vi "createFloat.vi"(8 "error in (no error)":errorcluster, 10 "Value":dbl, 11 "IInteger in":refnum<class "IFloat.lvclass">) -> (0 "error out":errorcluster, 3 "IInteger out":refnum<class "IFloat.lvclass">)   [LabVIEW 2022 SP3, in "openDAQ.lvlib" / "daqCoreTypes.lvlib" / "IFloat.lvclass"]
uses:
  <instrlib>/openDAQ/Public/Classes/daqCoreTypes/IFloat/IFloat.lvclass
  C:/Program Files (x86)/National Instruments/LabVIEW 2022/instr.lib/openDAQ/Public/Classes/IBaseObject/IBaseObject.lvclass
  <instrlib>/openDAQ/Public/Classes/IBaseObject/IBaseObject.lvclass/IBaseObject.ctl
  <instrlib>/openDAQ/Public/Classes/IBaseObject/Accessor/Read reference.vi
  <instrlib>/openDAQ/Public/Classes/IBaseObject/Accessor/Write reference.vi
  <instrlib>/openDAQ/Binaries/Windows/x86/copendaq32.dll
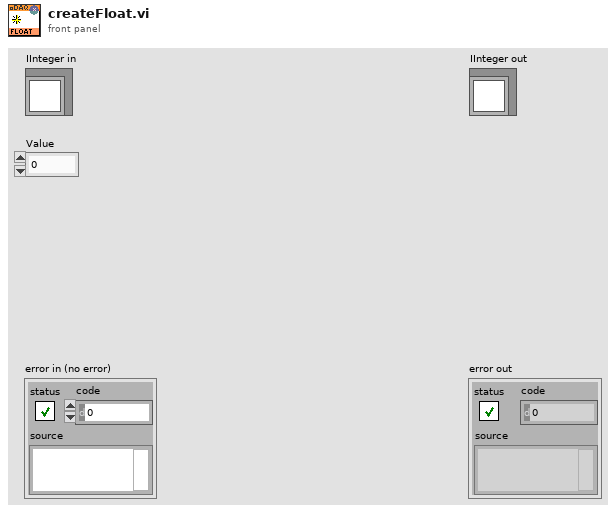
[diagram p1: front panel]
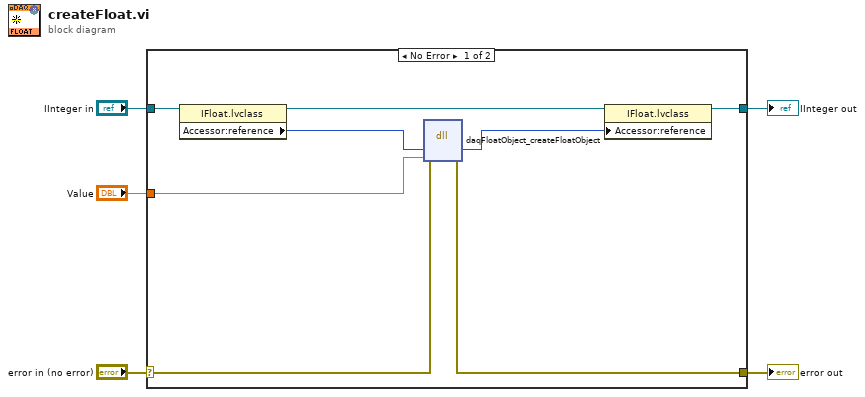
[diagram p0: block diagram]
diagram:
  n1 = case shown="No Error" "error in (no error)" {
    selector: "error in (no error)" -> [w12 w15]
    tunnel: [w11 w15] -> w4
    tunnel: [w9 w14] -> w2
    tunnel: "IInteger in" -> [w13 w14]
    tunnel: "Value" -> [w6 _]
    frame No Error {
      n2 = property class="IFloat.lvclass"(reference=w13) -> (reference out=w10:refnum<class "IFloat.lvclass">, "Accessor:reference"=w8:i64)  [unwired: 1 in, 1 out]
      n3 = dll-call lib="C:/Program Files (x86)/National Instruments/LabVIEW 2022/instr.lib/openDAQ/Binaries/Windows/x86/copendaq*.*" fn="daqFloatObject_createFloatObject"(error in=w12, "obj"=w8, "value"=w6) -> (error out=w11:errorcluster, "obj"=w7:i64)  [unwired: 4 in, 1 out]
      n4 = property class="IFloat.lvclass"(reference=w10, "Accessor:reference"=w7) -> (reference out=w9:refnum<class "IFloat.lvclass">)  [unwired: 1 in, 1 out]
    }
    frame Error {
    }
  }
  "error out" <- w4
  "IInteger out" <- w2
